vi "Bridge Balancing.vi"   [LabVIEW 2011]
uses:
  <vilib>/Rock Robotics/WPI/Relay/WPI_RelayValue.ctl
  System Set Points and States.vi
types:
  T1 = typedef "WPI_RelayValue.ctl" = enum16{"Off", "On", "Forward", "Reverse"}
  T2 = typedef "WPI_DigitalInputDevRef.ctl" = cluster{"DevStatus":errorcluster, "DIO Channel":T3, "Digital Module":T4}
  T3 = typedef "FPGA_DIOChannel.ctl" = enum8{"DIO 1", "DIO 2", "DIO 3", "DIO 4", "DIO 5", "DIO 6", "DIO 7", "DIO 8", "DIO 9", "DIO 10", "DIO 11", "DIO 12", "DIO 13", "DIO 14", "Invalid"}
  T4 = typedef "FPGA_TypedefDigitalModule.ctl" = enum16{"Digital Module 1", "Digital Module 2"}
  T5 = typedef "WPI_RelayDevRef.ctl" = cluster{"DevStatus":errorcluster, "Relay Channel":T6, "Digital Module":T4, "Relay Direction":T7}
  T6 = typedef "FPGA_DIORelayChannel.ctl" = enum8{"Relay 1", "Relay 2", "Relay 3", "Relay 4", "Relay 5", "Relay 6", "Relay 7", "Relay 8", "Invalid"}
  T7 = typedef "WPI_RelayDirection.ctl" = enum16{"Both directions", "Forward only", "Reverse only"}
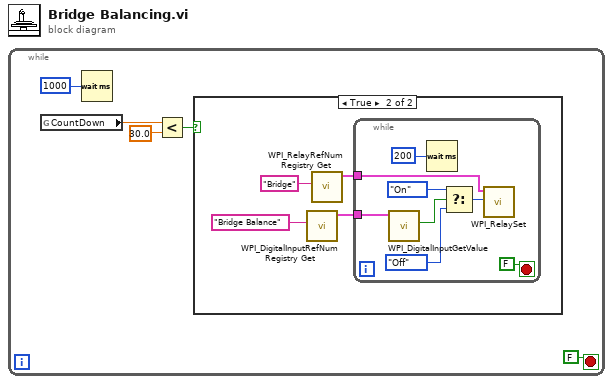
[diagram p0: block diagram]
diagram:
  n1 = while {
    stop <- FALSE stop-if-true
    n2 = global read "System Set Points and States.vi" "CountDown"() -> (w5:dbl)
    n3 = Wait (ms)(milliseconds to wait=u32 1000) -> ()  [unwired: 1 out]
    n4 = Less?(x=w5, y=30.0) -> (x < y?=w2:bool)
    n5 = case shown="True" w2 {
      frame False {
      }
      frame True {
        n6 = call <vilib>:"WPI_DigitalInputRefNum Registry Get.vi"("refnum name"="Bridge Balance") -> ("DigitalInputDevRef"=w6:T2)  [unwired: 9 in, 1 out]
        n7 = call <vilib>:"WPI_RelayRefNum Registry Get.vi"("refnum name"="Bridge") -> ("RelayDevRef"=w8:T5)  [unwired: 9 in, 1 out]
        n8 = while {
          tunnel: w8 -> [w16]
          tunnel: w6 -> [w17]
          stop <- FALSE stop-if-true
          n9 = call <vilib>:"WPI_DigitalInputGetValue.vi"("DigitalInputDevRef"=w17) -> ("Value"=w15:bool)  [unwired: 8 in, 2 out]
          n10 = Wait (ms)(milliseconds to wait=u32 200) -> ()  [unwired: 1 out]
          n11 = Select(t=WPI_RelayValue."On" ("RelayValue"), s=w15, f=WPI_RelayValue."Off" ("RelayValue")) -> (s? t:f=w12:T1)
          n12 = call <vilib>:"WPI_RelaySet.vi"("RelayValue"=w12, "RelayDevRef"=w16) -> ()  [unwired: 8 in, 2 out]
        }
      }
    }
  }
